vi "Logger Create Queue.vi"(0 "Queue Name":string, 11 "error in (no error)":errorcluster) -> (6 "File Ref Out":refnum<file>, 15 "error out":errorcluster)   [LabVIEW 2018]
uses:
  Logger Global.vi
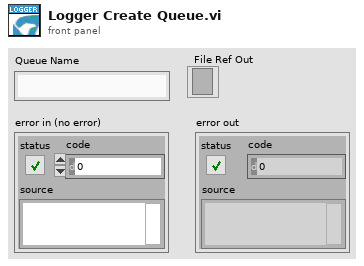
[diagram p1: front panel]
types:
  T1 = enum16{"open", "replace", "create", "open or create", "replace or create", "replace or create with confirmation"}
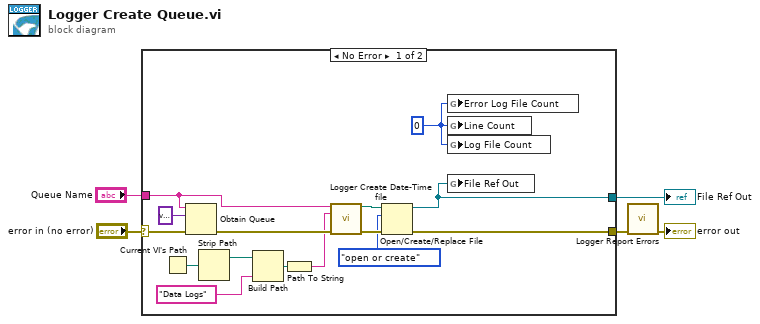
[diagram p0: block diagram]
diagram:
  n1 = case shown="No Error" "error in (no error)" {
    selector: "error in (no error)" -> [w20 w21]
    tunnel: [w16 w21] -> w4
    tunnel: "Queue Name" -> [w6 _]
    tunnel: [w13 _] -> w2
    frame No Error {
      w7 = u16 0 ("Log File Count")
      n2 = Current VI's Path() -> (path=w12:path)
      n3 = Obtain Queue(name (unnamed)=w6, element data type=variant, error in (no error)=w20) -> (error out=w18:errorcluster)  [unwired: 2 in, 2 out]
      n4 = Strip Path(path=w12) -> (stripped path=w11:path)  [unwired: 1 out]
      n5 = Build Path(base path=w11, name or relative path="Data Logs") -> (appended path=w9:path)
      n6 = Path To String(path=w9) -> (string=w8:string)
      n7 = call "Logger Create Date-Time file.vi"("File name"=w6, "Desired path"=w8, "error in (no error)"=w18) -> ("Path and name"=w14:path, "error out"=w17:errorcluster)  [unwired: 11 in]
      n8 = Open/Create/Replace File(file path (use dialog)=w14, error in=w17, operation (0:open)=T1."open or create") -> (refnum out=w13:refnum<file>, error out=w16:errorcluster)  [unwired: 3 in, 1 out]
      n9 = global write "Logger Global.vi" "Error Log File Count"(w7) -> ()
      n10 = global write "Logger Global.vi" "Line Count"(w7) -> ()
      n11 = global write "Logger Global.vi" "Log File Count"(w7) -> ()
      n12 = global write "Logger Global.vi" "File Ref Out"(w13) -> ()
    }
    frame Error {
    }
  }
  "File Ref Out" <- w2
  n13 = call "Logger Report Errors.vi"("error in (no error)"=w4) -> ("error out"=→"error out":errorcluster)  [unwired: 14 in]
